vi "MenuFixer.vi"(6 "Menu Name":string[](array[string]), 11 "Prefix":string) -> (5 "Item Tags":string[](array[string]), 7 "Item Names":string[](array[string]))   [LabVIEW 2011]
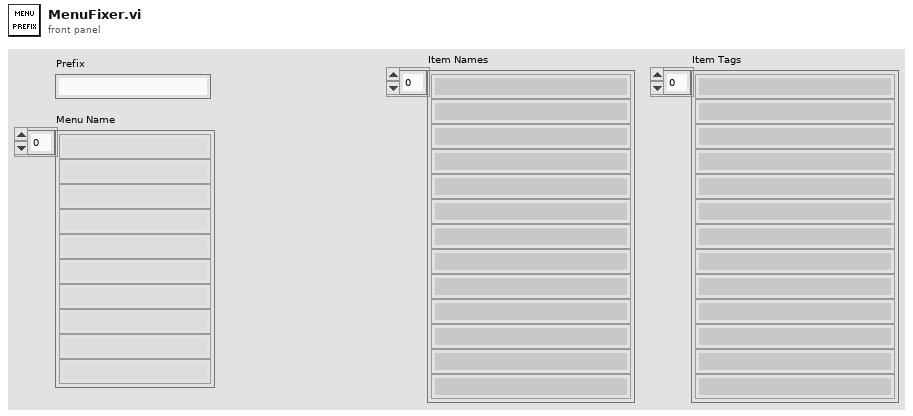
[diagram p1: front panel]
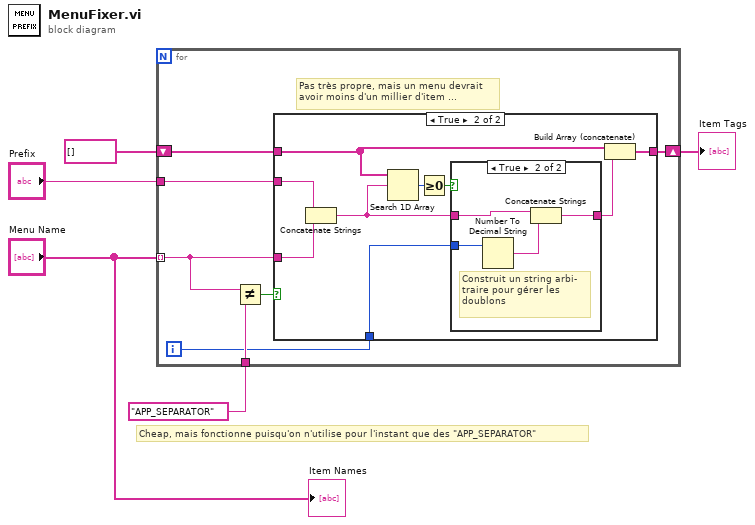
[diagram p0: block diagram]
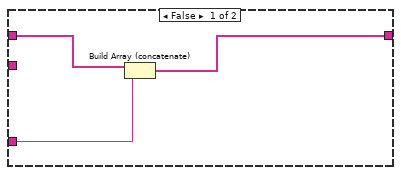
[diagram p2: hidden frame]
diagram:
  # "Cheap, mais fonctionne puisqu'on n'utilise pour l'instant que des \"APP_SEPARATOR\""
  n1 = for {
    tunnel: "Menu Name" -> [w9] mode=indexing
    tunnel: "Prefix" -> [w10]
    tunnel: "APP_SEPARATOR" -> [w12]
    shift-right: [w8] -> w3
    shift-left: string[] [] -> [w7]
    i -> [w6]
    # "Pas très propre, mais un menu devrait\navoir moins d'un millier d'item ..."
    n2 = Not Equal?(x=w9, y=w12) -> (x != y?=w11:bool)
    n3 = case shown="True" w11 {
      tunnel: w10 -> [_ w24]
      tunnel: w9 -> [w14 w23]
      tunnel: [w13 w22] -> w8
      tunnel: w7 -> [w15 w21]
      tunnel: w6 -> [_ w16]
      frame False {
        n4 = Build Array (concatenate)(w15, w14) -> (w13:string[])
      }
      frame True {
        n5 = Concatenate Strings(w24, w23) -> (w18:string)
        n6 = Search 1D Array(1D array=w21, element=w18) -> (index of element=w20:i32)  [unwired: 1 in]
        n7 = Greater Or Equal To 0?(x=w20) -> (x >= 0?=w19:bool)
        n8 = case shown="True" w19 {
          tunnel: [w25 w26] -> w17
          tunnel: w18 -> [w25 w28]
          tunnel: w16 -> [_ w29]
          frame False {
          }
          frame True {
            # "Construit un string arbi-\ntraire pour gérer les \ndoublons"
            n9 = Number To Decimal String(number=w29) -> (decimal integer string=w27:string)  [unwired: 1 in]
            n10 = Concatenate Strings(w28, w27) -> (w26:string)
          }
        }
        n11 = Build Array (concatenate)(w21, w17) -> (w22:string[])
      }
    }
  }
  "Item Tags" <- w3
  "Item Names" <- "Menu Name"
